vi "TimeStamp-Extractor.vi"(7 "TimeStampArray":dbl[](array[numeric]) format="%<%I:%M:%S%1u %p\n%Y/%m/%d>T") -> (4 "FirstTimestamp":dbl format="%<%I:%M:%S%1u %p\n%Y/%m/%d>T", 8 "Interval (sec)":dbl format="%.3f", 15 "LastTimestamp":dbl format="%<%I:%M:%S%1u %p\n%Y/%m/%d>T")   [LabVIEW 2011]
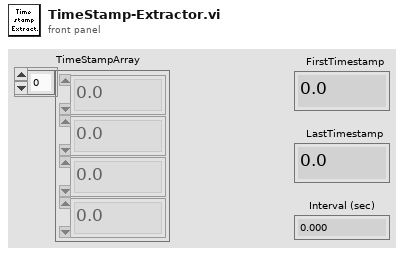
[diagram p1: front panel]
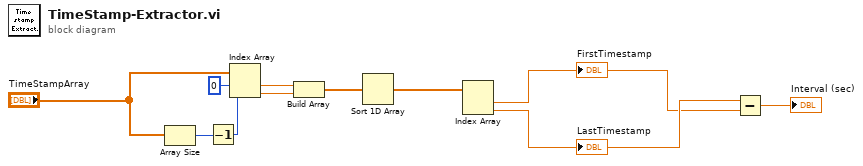
[diagram p0: block diagram]
diagram:
  n1 = Array Size(array="TimeStampArray") -> (size(s)=w10:i32)
  n2 = Decrement(x=w10) -> (x-1=w9:i32)
  n3 = Index Array(array="TimeStampArray", index #1=0 ("index"), index #2=w9) -> (element #1=w7:dbl, element #2=w8:dbl)
  n4 = Build Array(w7, w8) -> (w6:dbl[])
  n5 = Sort 1D Array(array=w6) -> (sorted array=w5:dbl[])
  n6 = Index Array(array=w5) -> (element #1=w3:dbl, element #2=w4:dbl)  [unwired: 2 in]
  "FirstTimestamp" <- w3
  "LastTimestamp" <- w4
  n7 = Subtract(x=w4, y=w3) -> (x-y=→"Interval (sec)":dbl)
